vi "Sys Config window globals.vi"() -> ()   [LabVIEW 2013]
uses:
  Typedefs/HW config window refs cluster.ctl
  Typedefs/HW Setup tab control.ctl
  Typedefs/DAQ FPGA config cluster.ctl
  RIG-SPECIFIC FILES/FPGA Refs/FPGA Ref.ctl
  <vilib>/userdefined/High Color/nirio_resource_hc.ctl
  Typedefs/FPGA input type AC-DC.ctl
  Peripherals Control/Triggers/Typedefs/Triggers output setup.ctl
  Peripherals Control/Triggers/Typedefs/Trigger setup element cluster.ctl
  Typedefs/AOL Properties Cluster.ctl
  Typedefs/CTRL system config cluster ref.ctl
  Typedefs/CTRL system config cluster.ctl
panel:
  in  "System Config Tab Control":T1
  out "Set tab page":bool
  out "Window is open":bool
  out "Bring to front":bool
  in  "System config window refs":T2
  # "<----Typedef"
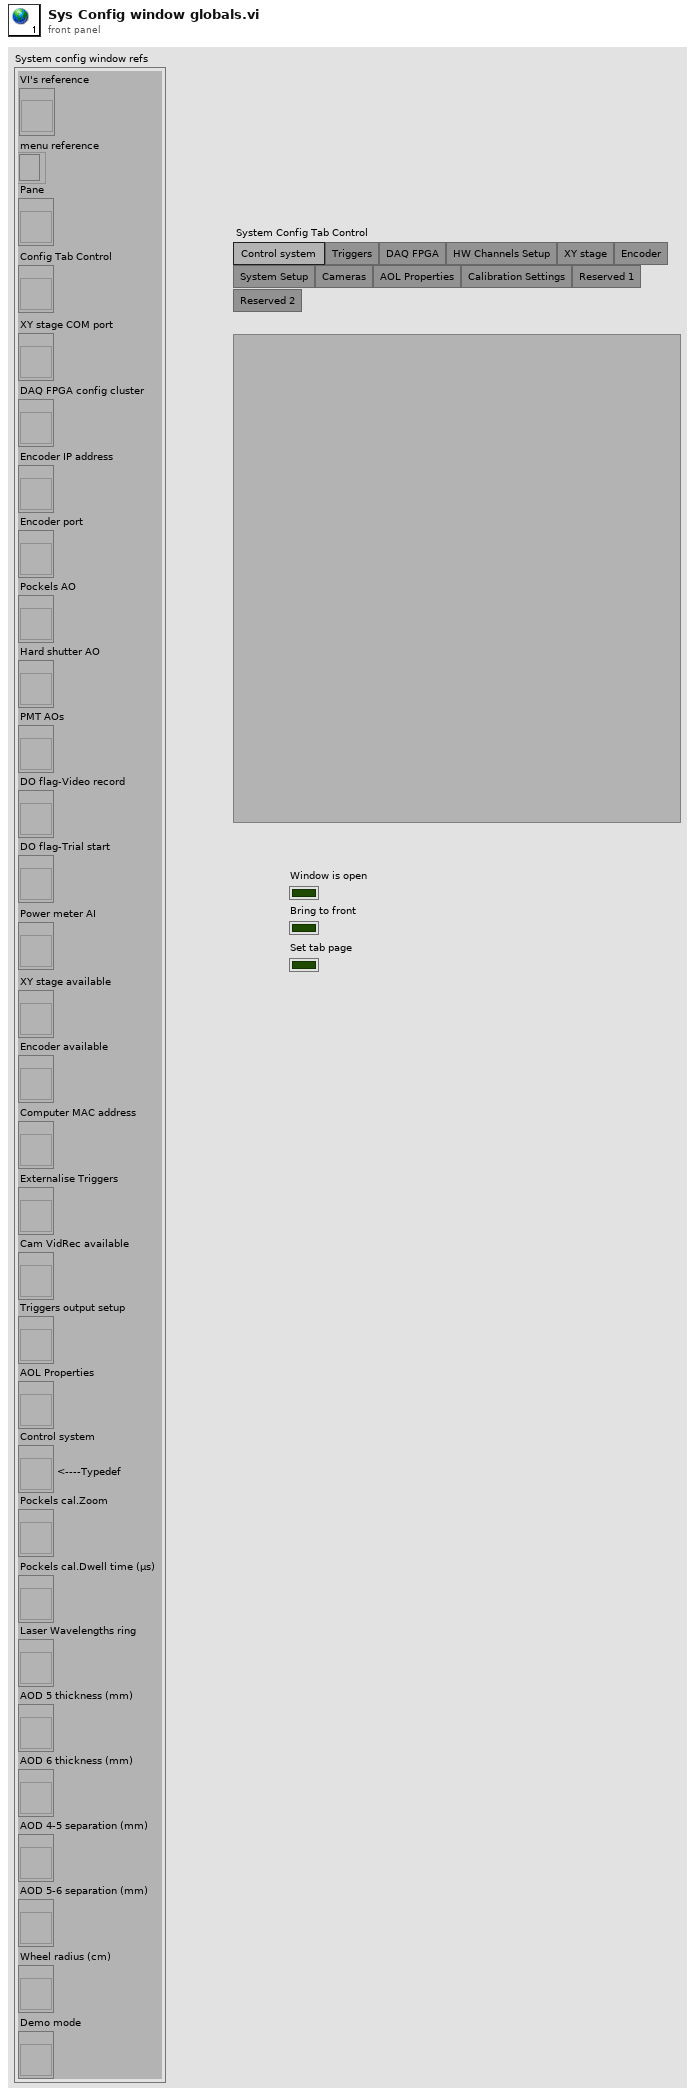
[diagram p1: front panel]
types:
  T1 = typedef "HW Setup tab control.ctl" = enum32{"Control system ", "Triggers", "DAQ FPGA", "HW Channels Setup", "XY stage", "Encoder", "System Setup", "Cameras", "AOL Properties", "Calibration Settings", "Reserved 1", "Reserved 2"}
  T2 = typedef "HW config window refs cluster.ctl" = cluster{"VI's reference":refnum<vi>, "menu reference":refnum<k9>, "Pane":refnum<vi>, "Config Tab Control":refnum<vi>, "XY stage COM port":refnum<vi>, "DAQ FPGA config cluster":refnum<vi>, "Encoder IP address":refnum<vi>, "Encoder port":refnum<vi>, "Pockels AO":refnum<vi>, "Hard shutter AO":refnum<vi>, "PMT AOs":refnum<vi>, "DO flag-Video record":refnum<vi>, "DO flag-Trial start":refnum<vi>, "Power meter AI":refnum<vi>, "XY stage available":refnum<vi>, "Encoder available":refnum<vi>, "Computer MAC address":refnum<vi>, "Externalise Triggers":refnum<vi>, "Cam VidRec available":refnum<vi>, "Triggers output setup":refnum<vi>, "AOL Properties":refnum<vi>, "Control system":T3, "Pockels cal.Zoom":refnum<vi>, "Pockels cal.Dwell time (µs)":refnum<vi>, "Laser Wavelengths ring":refnum<vi>, "AOD 5 thickness (mm)":refnum<vi>, "AOD 6 thickness (mm)":refnum<vi>, "AOD 4-5 separation (mm)":refnum<vi>, "AOD 5-6 separation (mm)":refnum<vi>, "Wheel radius (cm)":refnum<vi>, "Demo mode":refnum<vi>}
  T3 = typedef "CTRL system config cluster ref.ctl" = refnum<vi>
diagram:
